vi "Subdiagram Lables for Comments.vi"   [LabVIEW 2021]
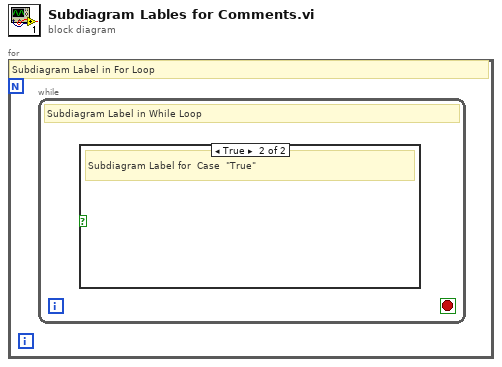
[diagram p0: block diagram]
diagram:
  n1 = for {
    # "Subdiagram Label in For Loop"
    n2 = while {
      stop <- _ stop-if-true
      # "Subdiagram Label in While Loop"
      n3 = case shown="True" {
        selector: _ -> [_ _]
        frame False {
        }
        frame True {
          # "Subdiagram Label for  Case  \"True\""
        }
      }
    }
  }
